vi "5.7.4-UDP Joystick Client.vi"() -> ()   [LabVIEW 2010]
doc: "This VI implements a client for the Named Service UDP Server.vi.\nIt connects to a service by specifying the server address and the name of the service. After sending a 'Hello' string to the server, the client receives the string sent by the server, displays the string and closes the connection.\n\n<b>Note:</b> This VI is built to work with the Named Service UDP Server.vi in UDP.llb."
uses:
  6-OCU Neurons/6.1-UDP Saitek.ctl
  5.0-Global.vi
panel:
  out "Joystick Data":T1 {"Right" scale=-32767.0..32767.0; "Left" scale=-32767.0..32767.0; "Yaw" scale=-32767.0..32767.0; "Roll" scale=-32767.0..32767.0; "Pitch" scale=-32767.0..32767.0}
  out "String":string
  out "error out":errorcluster
  in  "error in":errorcluster
  # "Instructions:\n1. Open Named Service UDP Server.vi located in the same library.\n2. Follow the instructions on it's front panel.\n\nNote: This VI is built to work with the Named Service UDP Server.vi in UDP.llb."
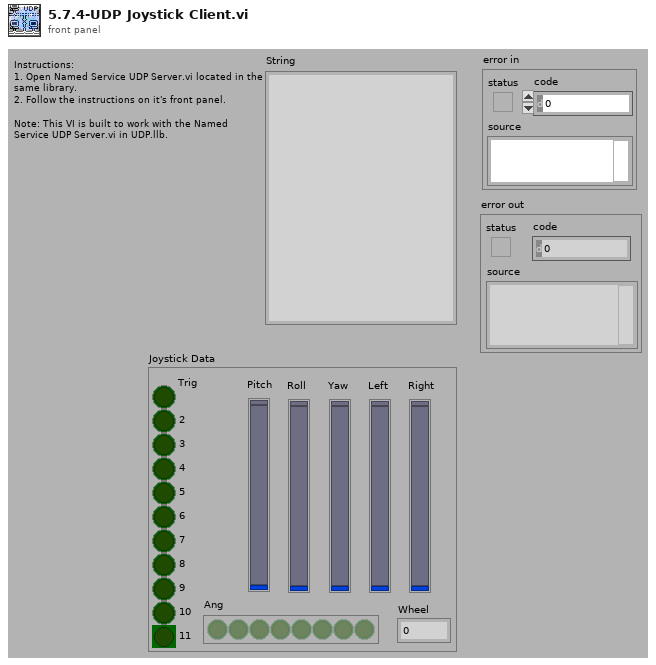
[diagram p1: front panel]
types:
  T1 = typedef "6.1-UDP Saitek.ctl" = cluster{"Trig":bool, "2":bool, "3":bool, "4":bool, "5":bool, "6":bool, "7":bool, "8":bool, "9":bool, "10":bool, "11":bool, "Pitch":i32, "Ang":bool[], "Wheel":dbl, "Roll":i32, "Yaw":i32, "Left":i32, "Right":i32}
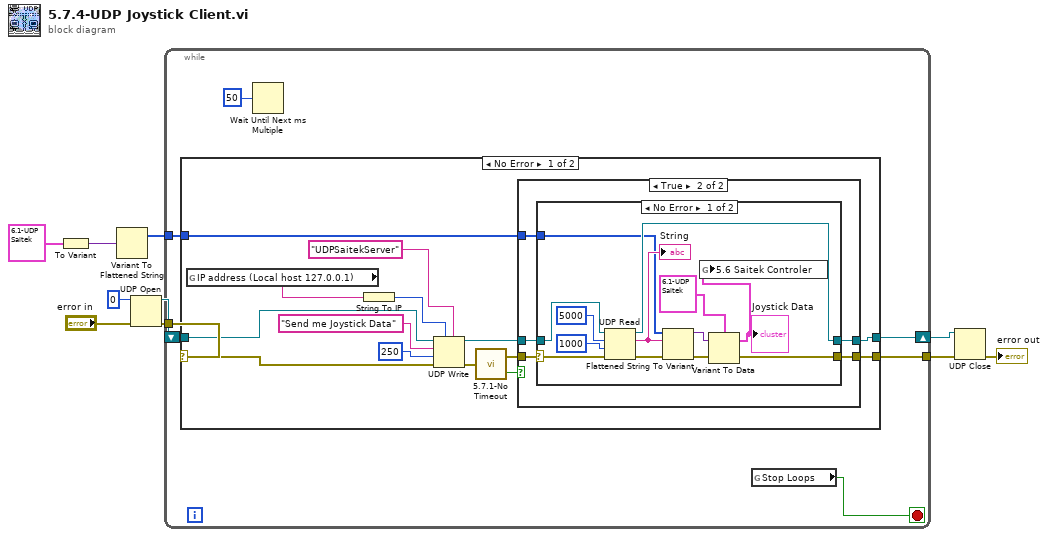
[diagram p0: block diagram]
diagram:
  n1 = To Variant(anything=T1 {"Trig"=FALSE, "2"=FALSE, "3"=FALSE, "4"=FALSE, "5"=FALSE, "6"=FALSE, "7"=FALSE, "8"=FALSE, "9"=FALSE, "10"=FALSE, "11"=FALSE, "Pitch"=0, "Ang"=[], "Wheel"=0.0, "Roll"=0, "Yaw"=0, "Left"=0, "Right"=0} ("Saitek Controler")) -> (Variant=w3:variant)
  n2 = Variant To Flattened String(Variant=w3) -> (1:w1:i16[])  [unwired: 1 out]
  n3 = UDP Open(8:"error in", 11:0) -> (port=w7:refnum<k16>, 0:w8:errorcluster)  [unwired: 3 in, 1 out]
  n4 = while {
    tunnel: [w17] -> w5
    tunnel: w8 -> [w16]
    shift-right: [w14] -> w6
    shift-left: w7 -> [w15]
    tunnel: w1 -> [w12]
    stop <- w11 stop-if-true
    n5 = case shown="No Error" w16 {
      selector: w16 -> [w31 w55]
      tunnel: [w26 w55] -> w17
      tunnel: w15 -> [w30 w54]
      tunnel: [w24 w54] -> w14
      tunnel: w12 -> [w19 _]
      frame No Error {
        n6 = global read "5.0-Global.vi" "IP address (Local host 127.0.0.1)"() -> (w18:string)
        n7 = String To IP(1:w18) -> (0:w29:u32)
        n8 = UDP Write(address=w29, port or service name="UDPSaitekServer", connection ID=w30, data in="Send me Joystick Data", 8:w31, 9:250 ("timeout ms (25000)")) -> (error out=w23:errorcluster, 3:w27:refnum<k16>)
        n9 = call "5.7.1-No Timeout.vi"("error in (no error)"=w23) -> ("No Timeout"=w21:bool, "error out"=w22:errorcluster)
        n10 = case shown="True" w21 {
          tunnel: w22 -> [w33 w38]
          tunnel: w27 -> [w32 w37]
          tunnel: [w32 w36] -> w24
          tunnel: [w33 w35] -> w26
          tunnel: w19 -> [_ w34]
          frame False {
          }
          frame True {
            n11 = case shown="No Error" w38 {
              selector: w38 -> [w51 w52]
              tunnel: w37 -> [w50 w53]
              tunnel: [w48 w53] -> w36
              tunnel: [w40 w52] -> w35
              tunnel: w34 -> [w45 _]
              frame No Error {
                n12 = UDP Read(connection ID=w50, max size (548)=5000, timeout ms (25000)=1000, 8:w51) -> (data out=w46:string, error out=w41:errorcluster, 3:w48:refnum<k16>)  [unwired: 2 out]
                "String" <- w46
                n13 = Flattened String To Variant(4:w41, 6:w46, 7:w45) -> (0:w42:errorcluster, 3:w44:variant)
                n14 = Variant To Data(error in=w42, Variant=w44, type=T1 {"Trig"=FALSE, "2"=FALSE, "3"=FALSE, "4"=FALSE, "5"=FALSE, "6"=FALSE, "7"=FALSE, "8"=FALSE, "9"=FALSE, "10"=FALSE, "11"=FALSE, "Pitch"=0, "Ang"=[], "Wheel"=0.0, "Roll"=0, "Yaw"=0, "Left"=0, "Right"=0} ("Saitek Controler")) -> (error out=w40:errorcluster, data=w39:T1)
                "Joystick Data" <- w39
                n15 = global write "5.0-Global.vi" "5.6 Saitek Controler"(w39) -> ()
              }
              frame Error {
              }
            }
          }
        }
      }
      frame Error {
      }
    }
    n16 = Wait Until Next ms Multiple(millisecond multiple=u32 50) -> ()  [unwired: 1 out]
    n17 = global read "5.0-Global.vi" "Stop Loops"() -> (w11:bool)
  }
  n18 = UDP Close(connection ID=w6, 8:w5) -> (error out=→"error out":errorcluster)  [unwired: 1 out]
